vi "Simulator Config Load Instruments.vi"(7 "Tree":refnum<vi>, 8 "error in (no error)":errorcluster, 10 "Port":u16=3388, 11 "IP":string="localhost" caption="Machine Location (IP / Fully Qualified Domain Name)") -> (0 "error out":errorcluster, 2 "Populated Configurations":T1[](array[typedef]) {"Calibration Date" format="%.2f"; "Parameters"."TX2pmax" format="%.1f"; "Parameters"."TX1pmax" format="%.1f"; "Parameters"."RXstop" format="%.1f"; "Parameters"."RXstart" format="%.1f"; "Parameters"."TX2stop" format="%.1f"; "Parameters"."TX2start" format="%.1f"; "Parameters"."TX1stop" format="%.1f"; "Parameters"."TX1start" format="%.1f"})   [LabVIEW 2011]
uses:
  PIM Configuration.ctl
  PIM Interface Language.ctl
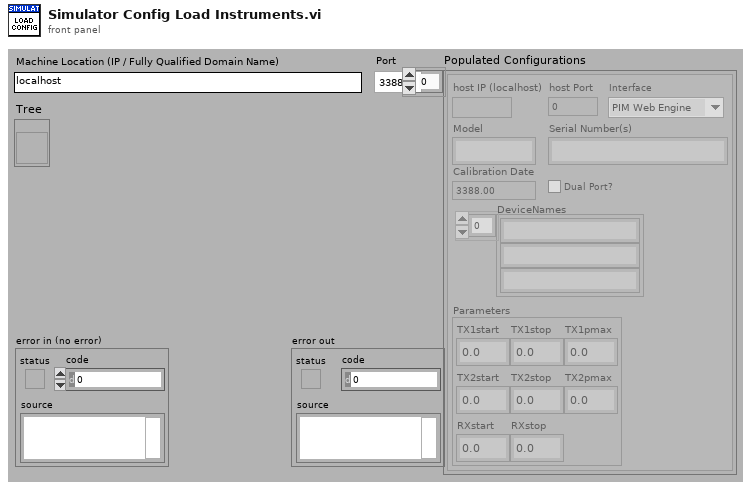
[diagram p1: front panel]
types:
  T1 = typedef "PIM Configuration.ctl" = cluster{"host IP (localhost)":string, "host Port":u16, "Model":string, "Serial Number(s)":string, "Calibration Date":dbl, "Dual Port?":bool, "DeviceNames":string[], "Parameters":cluster{"TX1start":dbl, "TX1stop":dbl, "TX1pmax":dbl, "TX2start":dbl, "TX2stop":dbl, "TX2pmax":dbl, "RXstart":dbl, "RXstop":dbl}, "Interface":T2}
  T2 = typedef "PIM Interface Language.ctl" = enum16{"PIM Web Engine", "PIM HW Engine"}
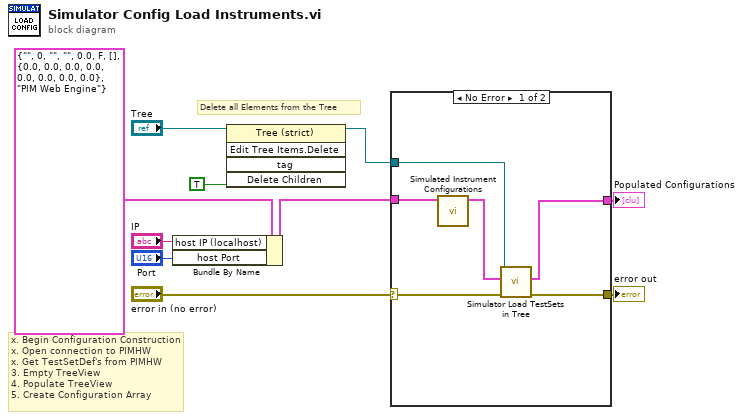
[diagram p0: block diagram]
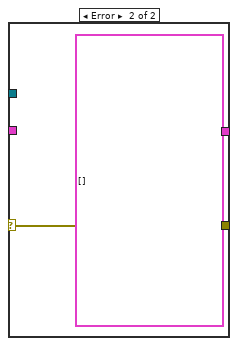
[diagram p2: hidden frame]
diagram:
  # "Delete all Elements from the Tree"
  # "x. Begin Configuration Construction\nx. Open connection to PIMHW\nx. Get TestSetDef's from PIMHW\n3. Empty TreeView\n4. Populate TreeView\n5. Create Configuration Array"
  n1 = Bundle By Name(cluster=T1 {"host IP (localhost)"="", "host Port"=0, "Model"="", "Serial Number(s)"="", "Calibration Date"=0.0, "Dual Port?"=FALSE, "DeviceNames"=[], "Parameters"={"TX1start"=0.0, "TX1stop"=0.0, "TX1pmax"=0.0, "TX2start"=0.0, "TX2stop"=0.0, "TX2pmax"=0.0, "RXstart"=0.0, "RXstop"=0.0}, "Interface"=enum."PIM Web Engine"} ("PIM Configuration"), "host IP (localhost)"="IP", "host Port"="Port") -> (w7:T1)
  n2 = invoke class="Tree (strict)" method="Edit Tree Items.Delete"(reference="Tree", "Delete Children"=TRUE ("Delete Children?")) -> (reference out=w4:refnum<vi>)  [unwired: 3 in, 4 out]
  n3 = case shown="No Error" "error in (no error)" {
    selector: "error in (no error)" -> [w12 w18]
    tunnel: [w13 w18] -> w1
    tunnel: w4 -> [w14 _]
    tunnel: w7 -> [w11 _]
    tunnel: [w16 T1[] [] ("Populated Configurations")] -> w6
    frame No Error {
      n4 = call "Simulated Instrument Configurations.vi"("Default Configuration"=w11) -> ("Simulation Configurations"=w15:T1[])  [unwired: 10 in]
      n5 = call "Simulator Load TestSets in Tree.vi"("error in (no error)"=w12, "Simulated Configurations"=w15, "Tree Control Reference"=w14) -> ("error out"=w13:errorcluster, "Populated Configurations"=w16:T1[])  [unwired: 7 in]
    }
    frame Error {
    }
  }
  "error out" <- w1
  "Populated Configurations" <- w6
